vi "capstone1 ver final.vi"() -> ()   [LabVIEW 2016]
uses:
  <instrlib>/Dynamixel Motor/Public/Motor Operation/Low Level/Baud Setting.ctl
  <vilib>/myRIO/Instrument Drivers/Onboard IO/DIO/typedefs/DIO Reference.ctl
  <vilib>/myRIO/Common/Instrument Driver Framework/Utilities/typedefs/myRIO Generic Hardware Reference.ctl
  <vilib>/myRIO/Common/Instrument Driver Framework/Utilities/typedefs/Hardware Version Enum.ctl
  <vilib>/myRIO/Common/Instrument Driver Framework/Utilities/typedefs/myRIO v1.0 Reference.ctl
  <vilib>/myRIO/Common/Instrument Driver Framework/Utilities/typedefs/Generic FPGA Reference.ctl
  <vilib>/myRIO/Common/Instrument Driver Framework/myRIO v1.0/DIO/typedefs/DIO Channels List.ctl
  <vilib>/myRIO/Common/Instrument Driver Framework/myRIO v1.0/DIO/typedefs/DIO Channels Enum.ctl
  <vilib>/userdefined/High Color/nirio_resource_hc.ctl
  <vilib>/myRIO/Instrument Drivers/Onboard IO/AI/typedefs/AI Reference.ctl
  <vilib>/myRIO/Common/Instrument Driver Framework/myRIO v1.0/AI/typedefs/AI Channels List.ctl
  <vilib>/myRIO/Common/Instrument Driver Framework/myRIO v1.0/AI/typedefs/AI Channels Enum.ctl
  <vilib>/myRIO/Common/Instrument Driver Framework/Utilities/typedefs/Analog Scaling Constants List.ctl
  <vilib>/myRIO/Common/Instrument Driver Framework/Utilities/typedefs/Analog Scaling Constants.ctl
  <vilib>/myRIO/Instrument Drivers/Onboard IO/AO/typedefs/AO Reference.ctl
  <vilib>/myRIO/Common/Instrument Driver Framework/myRIO v1.0/AO/typedefs/AO Channels List.ctl
  <vilib>/myRIO/Common/Instrument Driver Framework/myRIO v1.0/AO/typedefs/AO Channels Enum.ctl
  <vilib>/myRIO/Common/Instrument Driver Framework/Utilities/vis/Is FPGA Ref Available.vi
  <vilib>/myRIO/Common/Instrument Driver Framework/myRIO v1.0/DIO/vis/myRIO v1.1 Open DIO.vi
  <vilib>/myRIO/Instrument Drivers/Onboard IO/DIO/vis/Write.vi
  <vilib>/myRIO/Common/Instrument Driver Framework/myRIO v1.0/AI/vis/myRIO v1.1 Open AI.vi
  <vilib>/myRIO/Instrument Drivers/Onboard IO/AI/vis/Read.vi
  <vilib>/myRIO/Common/Instrument Driver Framework/myRIO v1.0/AO/vis/myRIO v1.1 Open AO.vi
  <vilib>/myRIO/Instrument Drivers/Onboard IO/AO/vis/Write.vi
  <vilib>/myRIO/Common/Instrument Driver Framework/Utilities/vis/Validate Channels.vi
  <vilib>/myRIO/Common/Instrument Driver Framework/myRIO v1.0/DIO/vis/myRIO v1.0 Reserve DIO.vi
  <vilib>/myRIO/Common/Instrument Driver Framework/myRIO v1.0/AI/vis/myRIO v1.0 Reserve AI.vi
  <vilib>/myRIO/Common/Instrument Driver Framework/myRIO v1.0/AO/vis/myRIO v1.0 Reserve AO.vi
  <vilib>/myRIO/Common/Instrument Driver Framework/myRIO v1.0/UART/vis/myRIO v1.0 Close UART.vi
  <vilib>/myRIO/Common/Instrument Driver Framework/myRIO v1.0/Resource Manager/vis/myRIO v1.0 Reserve Channel List.vi
  <vilib>/myRIO/Common/Instrument Driver Framework/myRIO v1.0/DIO/vis/myRIO v1.0 Build MUX Configuration DIO.vi
  <vilib>/myRIO/Common/Instrument Driver Framework/myRIO v1.0/AI/vis/myRIO v1.0 Build MUX Configuration AI.vi
  <vilib>/myRIO/Common/Instrument Driver Framework/myRIO v1.0/AO/vis/myRIO v1.0 Build MUX Configuration AO.vi
  <vilib>/myRIO/Common/Instrument Driver Framework/myRIO v1.0/Resource Manager/vis/myRIO v1.0 Reserve Channel.vi
  <vilib>/myRIO/Common/Instrument Driver Framework/myRIO v1.0/Resource Manager/vis/myRIO v1.0 Unreserve Channel.vi
  <vilib>/myRIO/Common/Instrument Driver Framework/myRIO v1.0/Resource Manager/vis/myRIO v1.0 Create Configuration List.vi
  <vilib>/myRIO/Common/Instrument Driver Framework/myRIO v1.0/Resource Manager/vis/myRIO v1.0 Build Mutex Name.vi
  <vilib>/Utility/VariantDataType/GetNumericInfo.vi
  <vilib>/Utility/error.llb/Error Cluster From Error Code.vi
  <vilib>/myRIO/Common/Instrument Driver Framework/myRIO v1.0/myRIO v1.1 Open.vi
  <vilib>/myRIO/Common/Instrument Driver Framework/Utilities/vis/IO Manager.vi
  <vilib>/myRIO/Common/Instrument Driver Framework/Utilities/vis/Configuration Manager.vi
  <vilib>/myRIO/Common/Instrument Driver Framework/myRIO v1.0/Resource Manager/vis/myRIO v1.0 Configure IO.vi
  <vilib>/myRIO/Common/Instrument Driver Framework/myRIO v1.0/myRIO v1.0 Close.vi
  <vilib>/myRIO/Common/Instrument Driver Framework/myRIO v1.0/DIO/vis/myRIO v1.0 Write DIO.vi
  <vilib>/myRIO/Common/Instrument Driver Framework/myRIO v1.0/AI/vis/myRIO v1.0 Get Scaling Constants AI.vi
  <vilib>/myRIO/Common/Instrument Driver Framework/myRIO v1.0/AI/vis/myRIO v1.0 Read AI.vi
  <vilib>/myRIO/Common/Instrument Driver Framework/myRIO v1.0/AO/vis/myRIO v1.0 Get Scaling Constants AO.vi
  <vilib>/myRIO/Common/Instrument Driver Framework/myRIO v1.0/AO/vis/myRIO v1.0 Write AO.vi
  <vilib>/myRIO/Common/Instrument Driver Framework/Utilities/vis/FPGA Ref Manager.vi
  <vilib>/myRIO/Common/Instrument Driver Framework/myRIO v1.0/myRIO v1.0 Reset FPGA.vi
  <vilib>/myRIO/Common/Instrument Driver Framework/myRIO v1.0/IRQ/vis/myRIO v1.0 IRQ Info FGV.vi
  <vilib>/myRIO/Common/Instrument Driver Framework/myRIO v1.0/IRQ/vis/myRIO v1.0 Timer IRQ Info FGV.vi
  <vilib>/myRIO/Common/Instrument Driver Framework/myRIO v1.0/IRQ/vis/myRIO v1.0 ISR Agent.vi
  <vilib>/myRIO/Express VI/Onboard Devices/LED/LED Express VI.xnode
  <vilib>/myRIO/Instrument Drivers/Onboard IO/DIO/vis/myRIO DIO Open.xnode
  <vilib>/myRIO/Express VI/Onboard IO/AI/AI Express VI.xnode
  <vilib>/myRIO/Instrument Drivers/Onboard IO/AI/vis/myRIO AI Open.xnode
  <vilib>/myRIO/Express VI/Onboard IO/AO/AO Express VI.xnode
  <vilib>/myRIO/Instrument Drivers/Onboard IO/AO/vis/myRIO AO Open.xnode
  <instrlib>/Dynamixel Motor/Dynamixel Motor.lvlib
  <vilib>/myRIO/Instrument Drivers/Onboard IO/DIO/DIO.lvlib
  <vilib>/myRIO/Instrument Drivers/Utilities/Utilities.lvlib
  <vilib>/myRIO/Instrument Drivers/Onboard IO/AO/AO.lvlib
  <vilib>/myRIO/Instrument Drivers/Onboard IO/AI/AI.lvlib
panel:
  out "temp cluster":T1
  in  "main stop":bool
  out "RT TCP Loop time":u32
  out "motor temp":cluster{"0":sgl, "1":sgl, "2":sgl, "3":sgl}
  out "value":T2
  out "TCP Read data":string
  in  "정지":bool
  out "error out":errorcluster
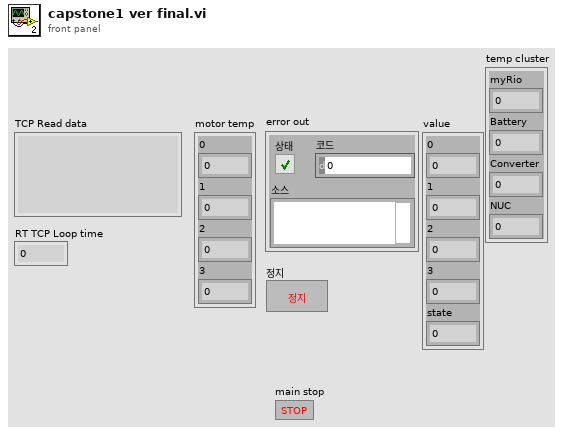
[diagram p1: front panel]
types:
  T1 = cluster{"myRio":dbl, "Battery":dbl, "Converter":dbl, "NUC":dbl}
  T2 = cluster{"0":sgl, "1":sgl, "2":sgl, "3":sgl, "state":sgl}
  T3 = typedef "DIO.lvlib/DIO Reference.ctl" = cluster{"myRIO Reference":T4, "DIO Channels List":T8}
  T4 = typedef "myRIO Generic Hardware Reference.ctl" = cluster{"myRIO Model":T5, "myRIO Hardware Reference":T6}
  T5 = typedef "Hardware Version Enum.ctl" = enum16{"Unknown", "myRIO-1900", "myRIO-1950", "roboRIO", "NI ELVIS RIO CM"}
  T6 = typedef "myRIO v1.0 Reference.ctl" = cluster{"Generic FPGA Reference":T7, "Allow multiple opens":bool}
  T7 = typedef "Generic FPGA Reference.ctl" = refnum<k20>
  T8 = typedef "DIO Channels List.ctl" = T9[]
  T9 = typedef "DIO Channels Enum.ctl" = enum16{"Not Connected", "C/DIO0", "C/DIO1", "C/DIO2", "C/DIO3", "C/DIO4", "C/DIO5", "C/DIO6", "C/DIO7", "A/DIO0", "A/DIO1", "A/DIO2", "A/DIO3", "A/DIO4", "A/DIO5", "A/DIO6", "A/DIO7", "A/DIO8", "A/DIO9", "A/DIO10", "A/DIO11", "A/DIO12", "A/DIO13", "A/DIO14", "A/DIO15", "B/DIO0", "B/DIO1", "B/DIO2", "B/DIO3", "B/DIO4", "B/DIO5", "B/DIO6", "B/DIO7", "B/DIO8", "B/DIO9", "B/DIO10", "B/DIO11", "B/DIO12", "B/DIO13", "B/DIO14", "B/DIO15", "LED0", "LED1", "LED2", "LED3", "Button0", "DIO/DIO0", "DIO/DIO1", "DIO/DIO2", "DIO/DIO3", "DIO/DIO4", "DIO/DIO5", "DIO/DIO6", "DIO/DIO7", "DIO/DIO8", "DIO/DIO9", "SPI/CS0", "SPI/CS1", "SPI/CS2", "SPI/CS3", "LED RADIO (Green)", "LED RADIO (Red)", "LED COMM (Green)", "LED COMM (Red)", "LED MODE (Green)", "LED MODE (Red)"}
  T10 = typedef "nirio_resource_hc.ctl" = tag
  T11 = cluster{"0":sgl, "1":sgl, "2":sgl, "3":sgl, "state":i32}
  T12 = typedef "AI.lvlib/AI Reference.ctl" = cluster{"myRIO Reference":T4, "AI Channels List":T13, "AI Scaling Constants List":T15}
  T13 = typedef "AI Channels List.ctl" = T14[]
  T14 = typedef "AI Channels Enum.ctl" = enum16{"Not Connected", "AudioIn/Left", "AudioIn/Right", "C/AI0", "C/AI1", "A/AI0", "A/AI1", "A/AI2", "A/AI3", "B/AI0", "B/AI1", "B/AI2", "B/AI3", "AI/AI0", "AI/AI1", "AI/AI2", "AI/AI3"}
  T15 = typedef "Analog Scaling Constants List.ctl" = T16[]
  T16 = typedef "Analog Scaling Constants.ctl" = cluster{"LSB Weight (Volts)":dbl, "Offset (Volts)":dbl, "Signed?":bool}
  T17 = typedef "AO.lvlib/AO Reference.ctl" = cluster{"myRIO Reference":T4, "AO Channel List":T18, "AO Scaling Constant List":T15}
  T18 = typedef "AO Channels List.ctl" = T19[]
  T19 = typedef "AO Channels Enum.ctl" = enum16{"Not Connected", "AudioOut/Left", "AudioOut/Right", "C/AO0", "C/AO1", "A/AO0", "A/AO1", "B/AO0", "B/AO1"}
  T20 = enum16{"big-endian, network order", "native, host order", "little-endian"}
  T21 = typedef "Dynamixel Motor.lvlib/Baud Setting.ctl" = u8
  T22 = cluster{"Temperature (C)":u8, "Temperature (C)":u8, "Temperature (C)":u8, "Temperature (C)":u8}
  T23 = cluster{"x/y":dbl, "x/y":dbl, "x/y":dbl, "x/y":dbl}
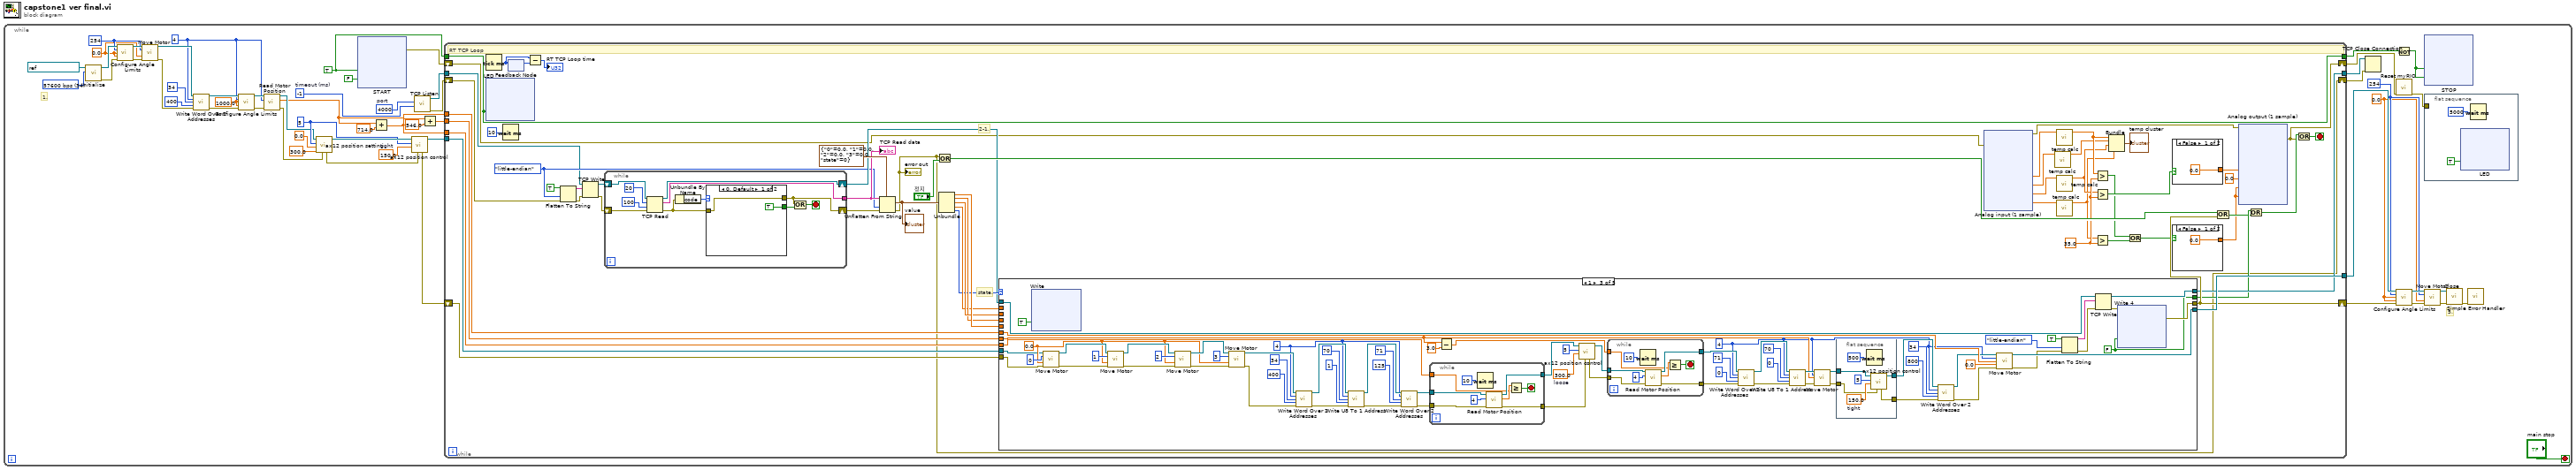
[diagram p0: block diagram]
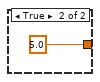
[diagram p2: hidden frame]
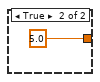
[diagram p3: hidden frame]
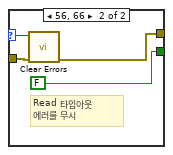
[diagram p4: hidden frame]
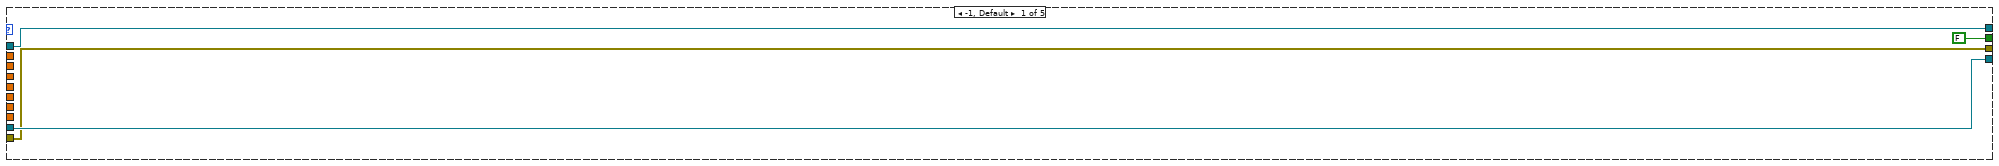
[diagram p5: hidden frame]
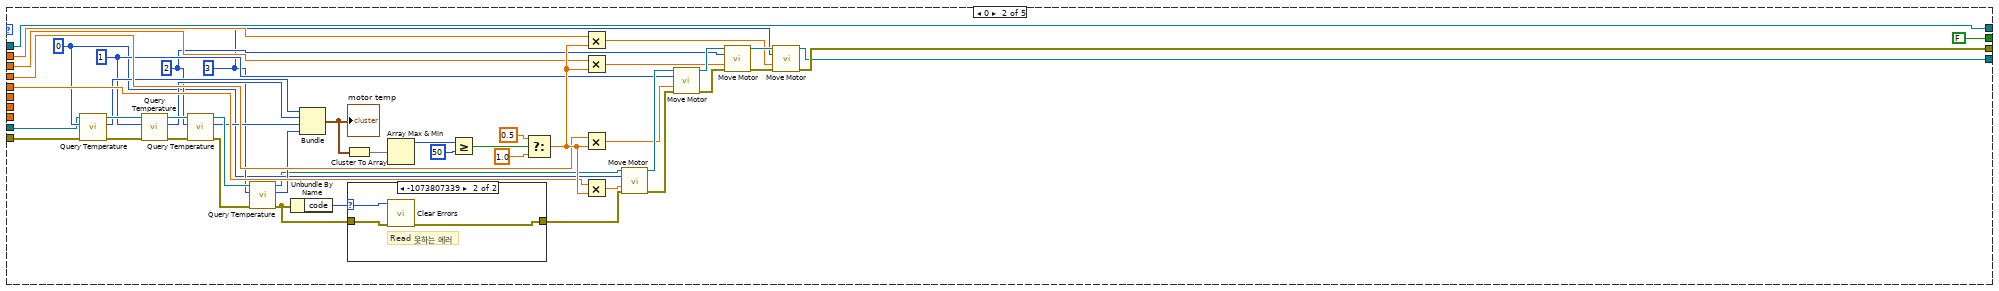
[diagram p6: hidden frame]
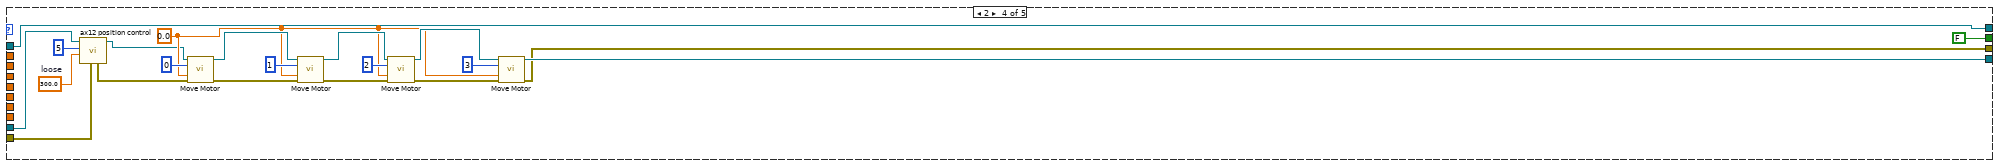
[diagram p8: hidden frame]
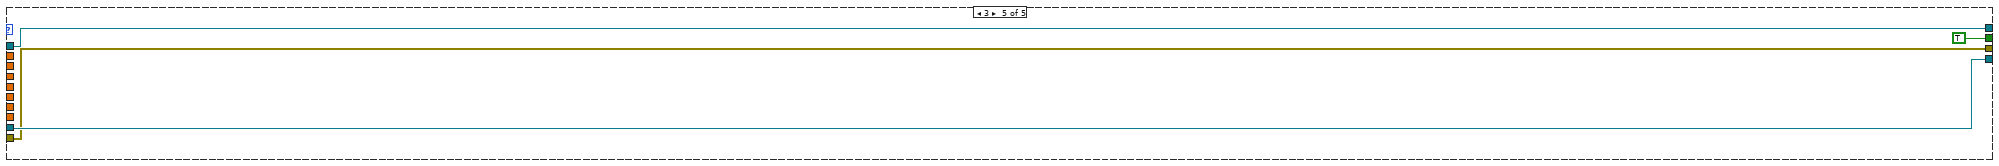
[diagram p9: hidden frame]
diagram:
  n1 = while {
    stop <- "main stop" stop-if-true
    w36 = 1000.0 ("Clockwise Angle Limit (0 deg)")
    w1 = 4
    w29 = 150.0  # tight
    w28 = 5
    w51 = T21 34 items=["1,000,000 bps"=1, "500,000 bps"=3, "400,000 bps"=4, "250,000 bps"=7, "200,000 bps"=9, "115200 bps"=16, "57600 bps"=34, "19200 bps"=103, "9600 bps"=207] ("Baud rate (57600 bps)")
    w41 = TRUE
    w22 = 0.0 ("Goal Speed (RPM)")
    w23 = u8 254 ("Motor ID (0)")
    w43 = u8 254 ("Motor ID (0)")
    w42 = 0.0 ("Clockwise Angle Limit (0 deg)")
    w55 = u16 4000  # port
    w56 = -1  # timeout (ms)
    # "5."
    # "1."
    n2 = call <instrlib>:"Initialize.vi"("Baud rate (57600 bps)"=w51, "VISA resource name"=refnum<visa-resource-name> "ASRL3::INSTR") -> ("error out"=w47:errorcluster, "VISA resource name out"=w46:refnum<visa-resource-name>)  [unwired: 8 in]
    n3 = call <instrlib>:"Configure Angle Limits.vi"("VISA resource name"=w46, "Motor ID (0)"=w43, "Clockwise Angle Limit (0 deg)"=w42, "Counter-Clockwise Angle Limit (300 deg)"=w42, "error in (no error)"=w47) -> ("VISA resource name out"=w45:refnum<visa-resource-name>, "error out"=w44:errorcluster)  [unwired: 9 in]
    n4 = call <instrlib>:"Move Motor.vi"("VISA resource name"=w45, "Motor ID (0)"=w43, "Goal Speed (RPM)"=w42, "error in (no error)"=w44) -> ("VISA resource name out"=w5:refnum<visa-resource-name>, "error out"=w4:errorcluster)  [unwired: 10 in]
    n5 = call <instrlib>:"Write Word Over 2 Addresses.vi"("VISA resource name"=w5, "Motor ID (0)"=w1, "Address number (0)"=u8 34, "Parameter (0)"=u16 400, "error in (no error)"=w4) -> ("VISA resource name out"=w2:refnum<visa-resource-name>, "error out"=w3:errorcluster)  [unwired: 9 in]
    n6 = call <instrlib>:"Configure Angle Limits.vi"("VISA resource name"=w2, "Motor ID (0)"=w1, "Clockwise Angle Limit (0 deg)"=w36, "Counter-Clockwise Angle Limit (300 deg)"=w36, "error in (no error)"=w3) -> ("VISA resource name out"=w21:refnum<visa-resource-name>, "error out"=w18:errorcluster)  [unwired: 9 in]
    n7 = call <instrlib>:"Read Motor Position.vi"("error in (no error)"=w18, "Motor ID (0)"=w1, "VISA resource name"=w21) -> ("error out"=w19:errorcluster, "Position (deg)"=w13:dbl, "VISA resource name out"=w20:refnum<visa-resource-name>)  [unwired: 6 in]
    n8 = call "ax12 position setting.vi"("error in (no error)"=w19, "Counter-Clockwise Angle Limit (300 deg)"=300.0 ("Clockwise Angle Limit (0 deg)"), "Clockwise Angle Limit (0 deg)"=0.0, "Motor ID (0)"=w28, "VISA resource name"=w20) -> ("VISA resource name out"=w33:refnum<visa-resource-name>, "error out"=w30:errorcluster)  [unwired: 5 in]
    n9 = xnode "START"("LED0"=w41, "LED3"=FALSE) -> ("error out"=w9:errorcluster)  [unwired: 1 in]
    n10 = Add(x=w13, y=714.0) -> (x+y=w14:dbl)
    n11 = call "ax12 position control.vi"("error in (no error)"=w30, "Goal Position (180 deg)"=w29, "Motor ID (0)"=w28, "VISA resource name"=w33) -> ("VISA resource name out"=w32:refnum<visa-resource-name>, "error out"=w31:errorcluster)  [unwired: 6 in]
    n12 = call <vilib>:"TCP Listen.vi"("timeout ms (wait forever: -1)"=w56, "port"=w55) -> ("error out"=w52:errorcluster, "connection ID"=w38:refnum<k5>)  [unwired: 5 in, 3 out]
    n13 = Add(x=w14, y=546.0) -> (x+y=w15:dbl)
    n14 = while {
      tunnel: w38 -> [w194]
      tunnel: [w202] -> w54
      shift-right: [w188] -> w53
      shift-left: w52 -> [w191]
      shift-right: [w211] -> w27
      shift-left: w31 -> [w210]
      tunnel: w41 -> [w219]
      tunnel: [w219] -> w49
      tunnel: [w212] -> w25
      tunnel: w32 -> [w204]
      tunnel: w15 -> [w201]
      tunnel: w14 -> [w200]
      tunnel: w13 -> [w199]
      shift-right: [w182] -> w8
      shift-left: w9 -> [w185]
      stop <- w181 stop-if-true
      w187 = 35.0 ("y")
      w195 = T20."little-endian" ("byte order (0:big-endian, network order)")
      # "state."
      # "2-1."
      # "RT TCP Loop"
      n15 = Tick Count (ms)() -> (millisecond timer value=w207:u32)
      n16 = xnode "LED"("LED1"=w219) -> ()  [unwired: 1 in, 1 out]
      n17 = Wait (ms)(milliseconds to wait=u32 10 ("대기 시간 (ms)")) -> ()  [unwired: 1 out]
      n18 = feedback #1() -> (w208:u32)  [unwired: 1 in]
      n19 = feedback-in #1(w207) -> ()
      n20 = Subtract(x=w207, y=w208) -> (x-y=→"RT TCP Loop time":u32)
      n21 = Flatten To String(anything=TRUE, byte order (0:big-endian, network order)=w195, error in (no error)=w191) -> (data string=w198:string, error out=w197:errorcluster)  [unwired: 1 in, 1 out]
      n22 = TCP Write(connection ID=w194, data in=w198, error in (no error)=w197) -> (connection ID out=w193:refnum<k5>, error out=w192:errorcluster)  [unwired: 1 in, 1 out]
      n23 = while {
        tunnel: [w316] -> w221
        shift-right: [w315] -> w203
        shift-left: w193 -> [w314]
        shift-right: [w310] -> w220
        shift-left: w192 -> [w313]
        stop <- w308 stop-if-true
        n24 = TCP Read(connection ID=w314, bytes to read=20 ("읽을 바이트"), error in (no error)=w313, 9:100 ("타임아웃 ms (25000)")) -> (connection ID out=w315:refnum<k5>, data out=w316:string, error out=w311:errorcluster)  [unwired: 1 in]
        n25 = Unbundle By Name(w311) -> ("code"=w312:i32)
        n26 = case shown="0, Default" w312 {
          selector: w312 -> [_ w323]
          tunnel: [w320 w322] -> w310
          tunnel: w311 -> [w320 w324]
          tunnel: [TRUE FALSE] -> w309
          frame 0, Default {
          }
          frame 56, 66 {
            # "Read 타임아웃\n에러를 무시"
            n27 = call <vilib>:"Clear Errors.vi"("error in (no error)"=w324, "specific error code to clear (0: all)"=w323) -> ("error out"=w322:errorcluster)  [unwired: 4 in, 1 out]
          }
        }
        n28 = Or(x=w310, y=w309) -> (x .or. y?=w308:bool)
      }
      "TCP Read data" <- w221
      n29 = Unflatten From String(type=T11 {"0"=0.0, "1"=0.0, "2"=0.0, "3"=0.0, "state"=0}, binary string=w221, byte order (0:big-endian, network order)=w195, error in (no error)=w220) -> (value=w218:T11, error out=w188:errorcluster)  [unwired: 1 in, 1 out]
      "error out" <- w188
      "value" <- w218
      n30 = Or(x=w188, y="정지") -> (x .or. y?=w209:bool)
      n31 = Unbundle(w218) -> ("0"=w217:sgl, "1"=w215:sgl, "2"=w216:sgl, "3"=w214:sgl, "state"=w213:i32)
      n32 = case shown="1" w213 {
        tunnel: w217 -> [_ w358 _ _ _]
        tunnel: w215 -> [_ w357 _ _ _]
        tunnel: w216 -> [_ w356 _ _ _]
        tunnel: w214 -> [_ w355 _ _ _]
        tunnel: [w328 w340 w429 w547 w568] -> w212
        tunnel: [w327 w341 w425 w546 w567] -> w211
        tunnel: w210 -> [w327 w338 w438 w552 w567]
        tunnel: w204 -> [w328 w331 w436 w551 w568]
        tunnel: w203 -> [w326 w330 w427 w554 w569]
        tunnel: [w326 w330 w428 w554 w569] -> w202
        tunnel: w201 -> [_ _ w394 _ _]
        tunnel: w200 -> [_ _ w420 _ _]
        tunnel: w199 -> [_ _ w424 _ _]
        tunnel: [FALSE FALSE w421 FALSE TRUE] -> w190
        frame -1, Default {
        }
        frame 0 {
          w342 = 3
          w343 = 2
          w344 = 1
          w339 = 0
          n33 = call <instrlib>:"Query Temperature.vi"("error in"=w338, "Motor ID (0)"=w339, "VISA resource name"=w331) -> ("error out"=w365:errorcluster, "Temperature (C)"=w354:u8, "VISA resource name out"=w368:refnum<visa-resource-name>)  [unwired: 6 in]
          n34 = call <instrlib>:"Query Temperature.vi"("error in"=w365, "Motor ID (0)"=w344, "VISA resource name"=w368) -> ("error out"=w364:errorcluster, "Temperature (C)"=w353:u8, "VISA resource name out"=w367:refnum<visa-resource-name>)  [unwired: 6 in]
          n35 = call <instrlib>:"Query Temperature.vi"("error in"=w364, "Motor ID (0)"=w343, "VISA resource name"=w367) -> ("error out"=w363:errorcluster, "Temperature (C)"=w352:u8, "VISA resource name out"=w366:refnum<visa-resource-name>)  [unwired: 6 in]
          n36 = call <instrlib>:"Query Temperature.vi"("error in"=w363, "Motor ID (0)"=w342, "VISA resource name"=w366) -> ("error out"=w345:errorcluster, "Temperature (C)"=w351:u8, "VISA resource name out"=w337:refnum<visa-resource-name>)  [unwired: 6 in]
          n37 = Unbundle By Name(w345) -> ("code"=w346:i32)
          n38 = Bundle("Temperature (C)"=w354, "Temperature (C)"=w353, "Temperature (C)"=w352, "Temperature (C)"=w351) -> (w348:T22)  [unwired: 1 in]
          "motor temp" <- w348
          n39 = Cluster To Array(cluster=w348) -> (array=w350:u8[])
          n40 = case shown="-1073807339" w346 {
            selector: w346 -> [_ w377]
            tunnel: [w375 w376] -> w336
            tunnel: w345 -> [w375 w378]
            frame 0, Default {
            }
            frame -1073807339 {
              # "Read 못하는 에러"
              n41 = call <vilib>:"Clear Errors.vi"("error in (no error)"=w378, "specific error code to clear (0: all)"=w377) -> ("error out"=w376:errorcluster)  [unwired: 4 in, 1 out]
            }
          }
          n42 = Array Max & Min(array=w350) -> (max value=w349:u8)  [unwired: 3 out]
          n43 = Greater Or Equal?(x=w349, y=50) -> (x >= y?=w347:bool)
          n44 = Select(t=0.5, s=w347, f=1.0) -> (s? t:f=w359:dbl)
          n45 = Multiply(x=w355, y=w359) -> (x*y=w332:dbl)
          n46 = Multiply(x=w356, y=w359) -> (x*y=w333:dbl)
          n47 = Multiply(x=w357, y=w359) -> (x*y=w334:dbl)
          n48 = Multiply(x=w358, y=w359) -> (x*y=w335:dbl)
          n49 = call <instrlib>:"Move Motor.vi"("VISA resource name"=w337, "Motor ID (0)"=w339, "Goal Speed (RPM)"=w335, "error in (no error)"=w336) -> ("VISA resource name out"=w369:refnum<visa-resource-name>, "error out"=w370:errorcluster)  [unwired: 10 in]
          n50 = call <instrlib>:"Move Motor.vi"("VISA resource name"=w369, "Motor ID (0)"=w344, "Goal Speed (RPM)"=w334, "error in (no error)"=w370) -> ("VISA resource name out"=w371:refnum<visa-resource-name>, "error out"=w373:errorcluster)  [unwired: 10 in]
          n51 = call <instrlib>:"Move Motor.vi"("VISA resource name"=w371, "Motor ID (0)"=w343, "Goal Speed (RPM)"=w333, "error in (no error)"=w373) -> ("VISA resource name out"=w372:refnum<visa-resource-name>, "error out"=w374:errorcluster)  [unwired: 10 in]
          n52 = call <instrlib>:"Move Motor.vi"("VISA resource name"=w372, "Motor ID (0)"=w342, "Goal Speed (RPM)"=w332, "error in (no error)"=w374) -> ("VISA resource name out"=w340:refnum<visa-resource-name>, "error out"=w341:errorcluster)  [unwired: 10 in]
        }
        frame 1 {
          w386 = 4
          w379 = 4
          w421 = FALSE ("notification")
          w433 = 300.0  # loose
          w439 = 0.0
          n53 = xnode "Write"("LED2"=TRUE) -> ()  [unwired: 1 in, 1 out]
          n54 = call <instrlib>:"Move Motor.vi"("VISA resource name"=w436, "Motor ID (0)"=0, "Goal Speed (RPM)"=w439, "error in (no error)"=w438) -> ("VISA resource name out"=w440:refnum<visa-resource-name>, "error out"=w441:errorcluster)  [unwired: 10 in]
          n55 = call <instrlib>:"Move Motor.vi"("VISA resource name"=w440, "Motor ID (0)"=1, "Goal Speed (RPM)"=w439, "error in (no error)"=w441) -> ("VISA resource name out"=w442:refnum<visa-resource-name>, "error out"=w444:errorcluster)  [unwired: 10 in]
          n56 = call <instrlib>:"Move Motor.vi"("VISA resource name"=w442, "Motor ID (0)"=2, "Goal Speed (RPM)"=w439, "error in (no error)"=w444) -> ("VISA resource name out"=w443:refnum<visa-resource-name>, "error out"=w445:errorcluster)  [unwired: 10 in]
          n57 = call <instrlib>:"Move Motor.vi"("VISA resource name"=w443, "Motor ID (0)"=3, "Goal Speed (RPM)"=w439, "error in (no error)"=w445) -> ("VISA resource name out"=w385:refnum<visa-resource-name>, "error out"=w382:errorcluster)  [unwired: 10 in]
          n58 = call <instrlib>:"Write Word Over 2 Addresses.vi"("VISA resource name"=w385, "Motor ID (0)"=w379, "Address number (0)"=u8 34, "Parameter (0)"=u16 400, "error in (no error)"=w382) -> ("VISA resource name out"=w384:refnum<visa-resource-name>, "error out"=w383:errorcluster)  [unwired: 9 in]
          n59 = call <instrlib>:"Write U8 To 1 Address.vi"("VISA resource name"=w384, "Motor ID (0)"=w379, "Address number (0)"=u8 70, "Parameter (0)"=u8 1, "error in (no error)"=w383) -> ("VISA resource name out"=w416:refnum<visa-resource-name>, "error out"=w415:errorcluster)  [unwired: 9 in]
          n60 = call <instrlib>:"Write Word Over 2 Addresses.vi"("VISA resource name"=w416, "Motor ID (0)"=w379, "Address number (0)"=u8 71, "Parameter (0)"=u16 125, "error in (no error)"=w415) -> ("VISA resource name out"=w414:refnum<visa-resource-name>, "error out"=w413:errorcluster)  [unwired: 9 in]
          n61 = while {
            tunnel: w414 -> [w503]
            tunnel: w413 -> [w502]
            tunnel: [w507] -> w435
            tunnel: [w506] -> w434
            tunnel: w420 -> [w505]
            stop <- w501 stop-if-true
            n62 = Wait (ms)(milliseconds to wait=u32 10 ("대기 시간 (ms)")) -> ()  [unwired: 1 out]
            n63 = call <instrlib>:"Read Motor Position.vi"("error in (no error)"=w502, "Motor ID (0)"=4, "VISA resource name"=w503) -> ("error out"=w506:errorcluster, "Position (deg)"=w508:dbl, "VISA resource name out"=w507:refnum<visa-resource-name>)  [unwired: 6 in]
            n64 = Greater Or Equal?(x=w508, y=w505) -> (x >= y?=w501:bool)
          }
          n65 = Subtract(x=w394, y=3.0) -> (x-y=w422:dbl)
          n66 = call "ax12 position control.vi"("error in (no error)"=w434, "Goal Position (180 deg)"=w433, "Motor ID (0)"=u8 5, "VISA resource name"=w435) -> ("VISA resource name out"=w431:refnum<visa-resource-name>, "error out"=w430:errorcluster)  [unwired: 6 in]
          n67 = while {
            tunnel: w431 -> [w493]
            tunnel: w430 -> [w494]
            tunnel: [w498] -> w400
            tunnel: [w497] -> w399
            tunnel: w422 -> [w496]
            stop <- w492 stop-if-true
            n68 = Wait (ms)(milliseconds to wait=u32 10 ("대기 시간 (ms)")) -> ()  [unwired: 1 out]
            n69 = call <instrlib>:"Read Motor Position.vi"("error in (no error)"=w494, "Motor ID (0)"=4, "VISA resource name"=w493) -> ("error out"=w497:errorcluster, "Position (deg)"=w499:dbl, "VISA resource name out"=w498:refnum<visa-resource-name>)  [unwired: 6 in]
            n70 = Greater Or Equal?(x=w499, y=w496) -> (x >= y?=w492:bool)
          }
          n71 = call <instrlib>:"Write Word Over 2 Addresses.vi"("VISA resource name"=w400, "Motor ID (0)"=w386, "Address number (0)"=u8 71, "Parameter (0)"=u16 0, "error in (no error)"=w399) -> ("VISA resource name out"=w405:refnum<visa-resource-name>, "error out"=w404:errorcluster)  [unwired: 9 in]
          n72 = call <instrlib>:"Write U8 To 1 Address.vi"("VISA resource name"=w405, "Motor ID (0)"=w386, "Address number (0)"=u8 70, "Parameter (0)"=u8 0, "error in (no error)"=w404) -> ("VISA resource name out"=w398:refnum<visa-resource-name>, "error out"=w397:errorcluster)  [unwired: 9 in]
          n73 = call <instrlib>:"Move Motor.vi"("VISA resource name"=w398, "Motor ID (0)"=w386, "Goal Position (180 deg)"=w394, "error in (no error)"=w397) -> ("VISA resource name out"=w396:refnum<visa-resource-name>, "error out"=w395:errorcluster)  [unwired: 10 in]
          n74 = flat-sequence {
            tunnel: w396 -> [w453]
            tunnel: w395 -> [w452]
            tunnel: [w451] -> w388
            tunnel: [w450] -> w390
            frame #0 {
              w454 = 150.0  # tight
              n75 = Wait (ms)(milliseconds to wait=u32 500) -> ()  [unwired: 1 out]
              n76 = call "ax12 position control.vi"("error in (no error)"=w452, "Goal Position (180 deg)"=w454, "Motor ID (0)"=u8 5, "VISA resource name"=w453) -> ("VISA resource name out"=w451:refnum<visa-resource-name>, "error out"=w450:errorcluster)  [unwired: 6 in]
            }
          }
          n77 = call <instrlib>:"Write Word Over 2 Addresses.vi"("VISA resource name"=w388, "Motor ID (0)"=w386, "Address number (0)"=u8 34, "Parameter (0)"=u16 800, "error in (no error)"=w390) -> ("VISA resource name out"=w387:refnum<visa-resource-name>, "error out"=w389:errorcluster)  [unwired: 9 in]
          n78 = call <instrlib>:"Move Motor.vi"("VISA resource name"=w387, "Motor ID (0)"=w386, "Goal Position (180 deg)"=w424, "Goal Speed (RPM)"=0.0, "error in (no error)"=w389) -> ("VISA resource name out"=w429:refnum<visa-resource-name>, "error out"=w409:errorcluster)  [unwired: 9 in]
          n79 = Flatten To String(anything=TRUE, byte order (0:big-endian, network order)=T20."little-endian", error in (no error)=w409) -> (data string=w411:string, error out=w410:errorcluster)  [unwired: 1 in, 1 out]
          n80 = TCP Write(connection ID=w427, data in=w411, error in (no error)=w410) -> (connection ID out=w428:refnum<k5>, error out=w426:errorcluster)  [unwired: 1 in, 1 out]
          n81 = xnode "Write 4"("LED2"=w421, "error in (no error)"=w426) -> ("error out"=w425:errorcluster)
        }
        frame 2 {
          w548 = 300.0  # loose
          w555 = 0.0
          n82 = call "ax12 position control.vi"("error in (no error)"=w552, "Goal Position (180 deg)"=w548, "Motor ID (0)"=5, "VISA resource name"=w551) -> ("VISA resource name out"=w550:refnum<visa-resource-name>, "error out"=w553:errorcluster)  [unwired: 6 in]
          n83 = call <instrlib>:"Move Motor.vi"("VISA resource name"=w550, "Motor ID (0)"=0, "Goal Speed (RPM)"=w555, "error in (no error)"=w553) -> ("VISA resource name out"=w565:refnum<visa-resource-name>, "error out"=w564:errorcluster)  [unwired: 10 in]
          n84 = call <instrlib>:"Move Motor.vi"("VISA resource name"=w565, "Motor ID (0)"=1, "Goal Speed (RPM)"=w555, "error in (no error)"=w564) -> ("VISA resource name out"=w563:refnum<visa-resource-name>, "error out"=w561:errorcluster)  [unwired: 10 in]
          n85 = call <instrlib>:"Move Motor.vi"("VISA resource name"=w563, "Motor ID (0)"=2, "Goal Speed (RPM)"=w555, "error in (no error)"=w561) -> ("VISA resource name out"=w562:refnum<visa-resource-name>, "error out"=w560:errorcluster)  [unwired: 10 in]
          n86 = call <instrlib>:"Move Motor.vi"("VISA resource name"=w562, "Motor ID (0)"=3, "Goal Speed (RPM)"=w555, "error in (no error)"=w560) -> ("VISA resource name out"=w547:refnum<visa-resource-name>, "error out"=w546:errorcluster)  [unwired: 10 in]
        }
        frame 3 {
        }
      }
      n87 = xnode "Analog input (1 sample)"("error in (no error)"=w185) -> ("Myrio (A/AI0 (Pin 3))"=w180:dbl, "Battery (A/AI1 (Pin 5))"=w172:dbl, "Converter (B/AI0 (Pin 3))"=w179:dbl, "NUC (B/AI1 (Pin 5))"=w178:dbl, "error out"=w184:errorcluster)
      n88 = call "temp calc.vi"("Numeric"=w172) -> ("x/y"=w170:dbl)  [unwired: 10 in]
      n89 = call "temp calc.vi"("Numeric"=w180) -> ("x/y"=w171:dbl)  [unwired: 10 in]
      n90 = call "temp calc.vi"("Numeric"=w179) -> ("x/y"=w169:dbl)  [unwired: 10 in]
      n91 = call "temp calc.vi"("Numeric"=w178) -> ("x/y"=w168:dbl)  [unwired: 10 in]
      n92 = Greater?(x=w171, y=w187) -> (0:w176:bool)
      n93 = Greater?(x=w169, y=w187) -> (0:w186:bool)
      n94 = Greater?(x=w168, y=w187) -> (0:w175:bool)
      n95 = Bundle("x/y"=w171, "x/y"=w170, "x/y"=w169, "x/y"=w168) -> (→"temp cluster":T23)  [unwired: 1 in]
      n96 = Or(x=w176, y=w175) -> (x .or. y?=w174:bool)
      n97 = case shown="False" w186 {
        tunnel: [0.0 5.0] -> w177
        frame False {
        }
        frame True {
        }
      }
      n98 = case shown="False" w174 {
        tunnel: [0.0 5.0] -> w173
        frame False {
        }
        frame True {
        }
      }
      n99 = Or(x=w209, y=w211) -> (x .or. y?=w189:bool)
      n100 = xnode "Analog output (1 sample)"("A/AO0 (Pin 2)"=w177, "A/AO1 (Pin 4)"=0.0, "B/AO0 (Pin 2)"=w173, "B/AO1 (Pin 4)"=w173, "error in (no error)"=w184) -> ("error out"=w182:errorcluster)
      n101 = Or(x=w190, y=w189) -> (x .or. y?=w183:bool)
      n102 = Or(x=w183, y=w182) -> (x .or. y?=w181:bool)
    }
    n103 = TCP Close Connection(connection ID=w54, error in (no error)=w53) -> ()  [unwired: 3 out]
    n104 = Not(x=w49) -> (.not. x?=w48:bool)
    n105 = call <vilib>:"Reset myRIO.vi"("error in (no error)"=w8) -> ("error out"=w12:errorcluster)  [unwired: 10 in]
    n106 = call <instrlib>:"Configure Angle Limits.vi"("VISA resource name"=w25, "Motor ID (0)"=w23, "Clockwise Angle Limit (0 deg)"=w22, "Counter-Clockwise Angle Limit (300 deg)"=w22, "error in (no error)"=w27) -> ("VISA resource name out"=w24:refnum<visa-resource-name>, "error out"=w26:errorcluster)  [unwired: 9 in]
    n107 = xnode "STOP"("LED0"=w48, "LED1"=w48) -> ()  [unwired: 1 in, 1 out]
    n108 = flat-sequence {
      tunnel: w12 -> [_]
      frame #0 {
        n109 = xnode "LED"("LED3"=TRUE) -> ()  [unwired: 1 in, 1 out]
        n110 = Wait (ms)(milliseconds to wait=5000) -> ()  [unwired: 1 out]
      }
    }
    n111 = call <instrlib>:"Move Motor.vi"("VISA resource name"=w24, "Motor ID (0)"=w23, "Goal Speed (RPM)"=w22, "error in (no error)"=w26) -> ("VISA resource name out"=w40:refnum<visa-resource-name>, "error out"=w39:errorcluster)  [unwired: 10 in]
    n112 = call <instrlib>:"Close.vi"("error in (no error)"=w39, "VISA resource name"=w40) -> ("error out"=w37:errorcluster)  [unwired: 9 in]
    n113 = call <vilib>:"Simple Error Handler.vi"("error in (no error)"=w37) -> ()  [unwired: 4 in, 5 out]
  }
